vi "Decide next action.vi"(7 "Polarization-based seek? (F)":bool, 8 "error in (no error)":errorcluster, 9 "\"Good\" rate threshold":dbl, 10 "Seek positive polarization?":bool, 11 "Automatic Mode in":refnum<class "Automatic Mode.lvclass">) -> (0 "error out":errorcluster, 1 "Calculated rate":dbl, 2 "Decision":T1, 3 "Automatic Mode out":refnum<class "Automatic Mode.lvclass">, 4 "Should reseek?":bool)   [LabVIEW 2019, in "Automatic Mode.lvclass"]
uses:
  Automatic Mode.lvclass
  Controller decision.ctl
  Automatic Mode.lvclass/Automatic Mode.ctl
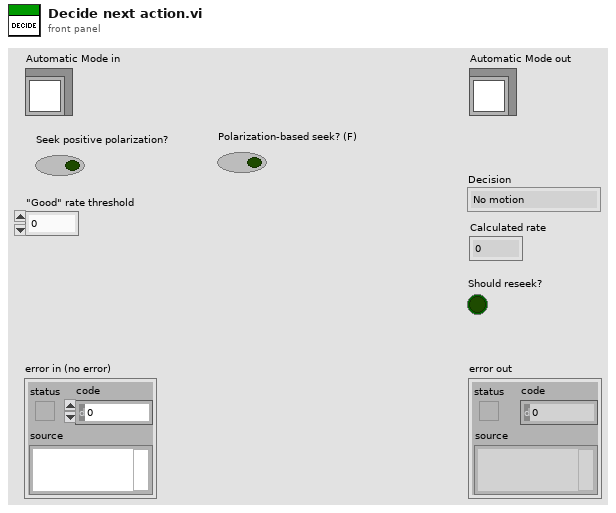
[diagram p1: front panel]
types:
  T1 = typedef "Controller decision.ctl" = enum16{"No motion", "Switch direction", "Keep current direction"}
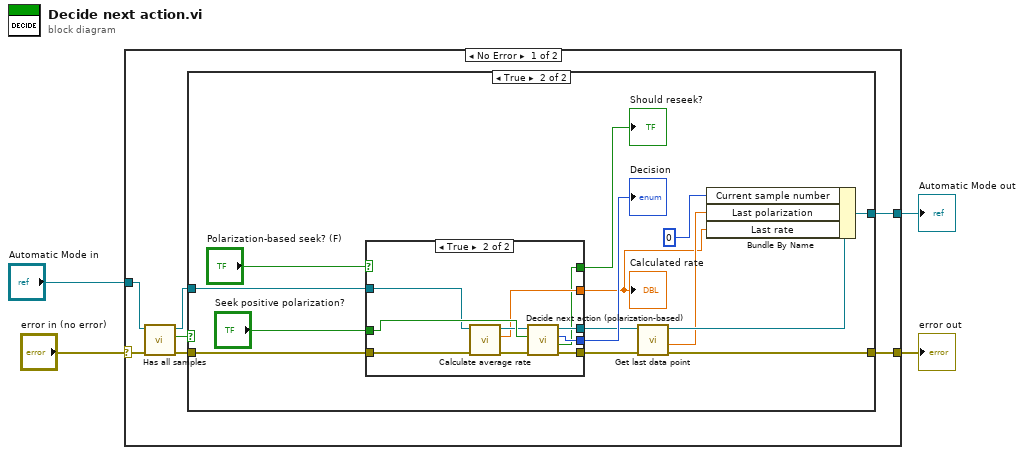
[diagram p0: block diagram]
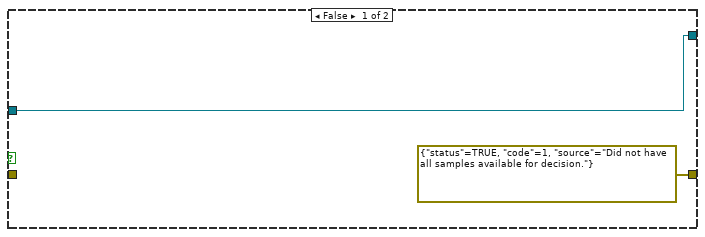
[diagram p2: hidden frame]
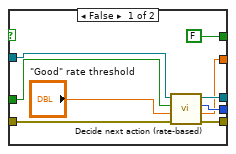
[diagram p3: hidden frame]
diagram:
  n1 = case shown="No Error" "error in (no error)" {
    selector: "error in (no error)" -> [w9 w48]
    tunnel: [w7 w48] -> w3
    tunnel: [w5 w47] -> w1
    tunnel: "Automatic Mode in" -> [w11 w47]
    frame No Error {
      n2 = call "Has all samples.vi"("error in (no error)"=w9, "Automatic Mode in"=w11) -> ("error out"=w8:errorcluster, "Has all samples?"=w10:bool, "Automatic Mode out"=w6:refnum<class "Automatic Mode.lvclass">)  [unwired: 7 in]
      n3 = case shown="True" w10 {
        tunnel: w8 -> [_ w16]
        tunnel: [errorcluster {"status"=TRUE, "code"=1, "source"="Did not have all samples available for decision."} ("error out") w19] -> w7
        tunnel: w6 -> [w12 w17]
        tunnel: [w12 w27] -> w5
        frame False {
        }
        frame True {
          n4 = case shown="True" "Polarization-based seek? (F)" {
            tunnel: w17 -> [w35 w39]
            tunnel: w16 -> [w36 w42]
            tunnel: "Seek positive polarization?" -> [w29 w46]
            tunnel: [w34 w45] -> w22
            tunnel: [w33 w44] -> w23
            tunnel: [w31 w43] -> w20
            tunnel: [w32 w38] -> w15
            tunnel: [FALSE w37] -> w14
            frame False {
              n5 = call "Decide next action (rate-based).vi"("error in (no error)"=w36, "\"Good\" rate threshold"="\"Good\" rate threshold", "Seek positive polarization?"=w29, "Automatic Mode in"=w35) -> ("error out"=w31:errorcluster, "New rate"=w32:dbl, "Decision"=w33:T1, "Automatic Mode out"=w34:refnum<class "Automatic Mode.lvclass">)  [unwired: 4 in]
            }
            frame True {
              n6 = call "Calculate average rate.vi"("error in (no error)"=w42, "Automatic Mode in"=w39) -> ("error out"=w41:errorcluster, "Average rate"=w38:dbl, "Automatic Mode out"=w40:refnum<class "Automatic Mode.lvclass">)  [unwired: 7 in]
              n7 = call "Decide next action (polarization-based).vi"("error in (no error)"=w41, "Seek positive polarization?"=w46, "Automatic Mode in"=w40) -> ("error out"=w43:errorcluster, "Should reseek?"=w37:bool, "Decision"=w44:T1, "Automatic Mode out"=w45:refnum<class "Automatic Mode.lvclass">)  [unwired: 5 in]
            }
          }
          "Decision" <- w23
          "Calculated rate" <- w15
          "Should reseek?" <- w14
          n8 = call "Get last data point.vi"("error in (no error)"=w20, "Automatic Mode in"=w22) -> ("error out"=w19:errorcluster, "Polarization"=w18:dbl, "Automatic Mode out"=w21:refnum<class "Automatic Mode.lvclass">)  [unwired: 6 in, 1 out]
          n9 = Bundle By Name(cluster=w21, "Current sample number"=0, "Last polarization"=w18, "Last rate"=w15) -> (w27:refnum<class "Automatic Mode.lvclass">)
        }
      }
    }
    frame Error {
    }
  }
  "error out" <- w3
  "Automatic Mode out" <- w1
